vi "initialize.vi"() -> (0 "ErrorOut":errorcluster, 3 "Queues":T1)   [LabVIEW 2019]
uses:
  utilities/Queues.ctl
  GUIVIs/GUIOutput.ctl
  masterVIs/Command.ctl
  MobileAnalyzer/mainVIs/analyzeAccelerationDataVIs/AccelerationDataFrames.ctl
  MobileAnalyzer/mainVIs/analyzeAccelerationDataVIs/AnalyzedVibrationsData.ctl
  MobileAnalyzer/mainVIs/analyzeAccelerationDataVIs/calculateFaultIndicatorsVIs/FaultDetections.ctl
  MobileAnalyzer/mainVIs/analyzeAccelerationDataVIs/calculateFaultIndicatorsVIs/FaultParameter.ctl
  MobileAnalyzer/mainVIs/analyzeAccelerationDataVIs/calculateFaultIndicatorsVIs/AxesValueAndFaultDetection.ctl
  utilities/DesktopAppSettings.ctl
  masterVIs/Thread.ctl
  MobileAnalyzer/mainVIs/analyzeAccelerationDataVIs/calculateFaultIndicatorsVIs/Thresholds.ctl
  MobileAnalyzer/mainVIs/utilities/FGVAction.ctl
  DialogsVIs/FilePathToSaveAction.ctl
  masterVIs/CommandQueuesAction.ctl
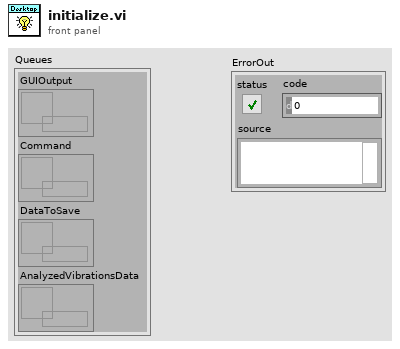
[diagram p1: front panel]
types:
  T1 = typedef "Queues.ctl" = cluster{"GUIOutput":refnum<queue>, "Command":refnum<queue>, "DataToSave":refnum<queue>, "AnalyzedVibrationsData":refnum<queue>}
  T2 = typedef "AnalyzedVibrationsData.ctl" = cluster{"AccelerationDataFrames":T3, "Fault detections":T4}
  T3 = typedef "AccelerationDataFrames.ctl" = cluster{"AccelerationData":waveform(dbl)[], "Amplitudes":cluster{"f0":dbl, "df":dbl, "real part":dbl[]}[], "Phases":cluster{"f0":dbl, "df":dbl, "imaginary part":dbl[]}[]}
  T4 = typedef "FaultDetections.ctl" = cluster{"Parameters labels":T5[], "Parameters fault detection":T6[], "Frequencies fault detection":T6[]}
  T5 = typedef "FaultParameter.ctl" = enum16{"Kurtosis", "RMS"}
  T6 = typedef "AxesValueAndFaultDetection.ctl" = cluster{"Axes Values":dbl[], "Axes Fault Detection":bool[]}
  T7 = typedef "Command.ctl" = enum16{"None", "Connect", "Start", "Stop", "RestartAnalyzer", "Exit", "OpenDataFile", "CanBegin", "FileToSaveSettings", "SetThresholds"}
  T8 = typedef "FilePathToSaveAction.ctl" = enum16{"Build new path", "Update index", "Get file path", "Get current settings"}
  T9 = typedef "FGVAction.ctl" = enum16{"Read", "Write"}
  T10 = typedef "CommandQueuesAction.ctl" = enum16{"Initialize", "Set", "Get", "ReleaseAll"}
  T11 = typedef "GUIOutput.ctl" = cluster{"Aquiring data":bool, "AnalyzerError":errorcluster, "FIFO overflow":bool, "Analyzing data":bool, "Connected":bool}
  T12 = typedef "Thread.ctl" = enum16{"GUI", "communicateWithAnalyzer", "saveDataToTDMS"}
  T13 = typedef "DesktopAppSettings.ctl" = cluster{"MobileAnalyzer IP":string, "Network Stream Timeout Code":i32, "Endpoint Destroyed Code":i32, "Save to file?":bool, "All threads":T12[], "Fault Thresholds":T14}
  T14 = typedef "Thresholds.ctl" = cluster{"Parameters labels":T5[], "Parameters thresholds":dbl[], "Freqs and thresholds":dbl[][]}
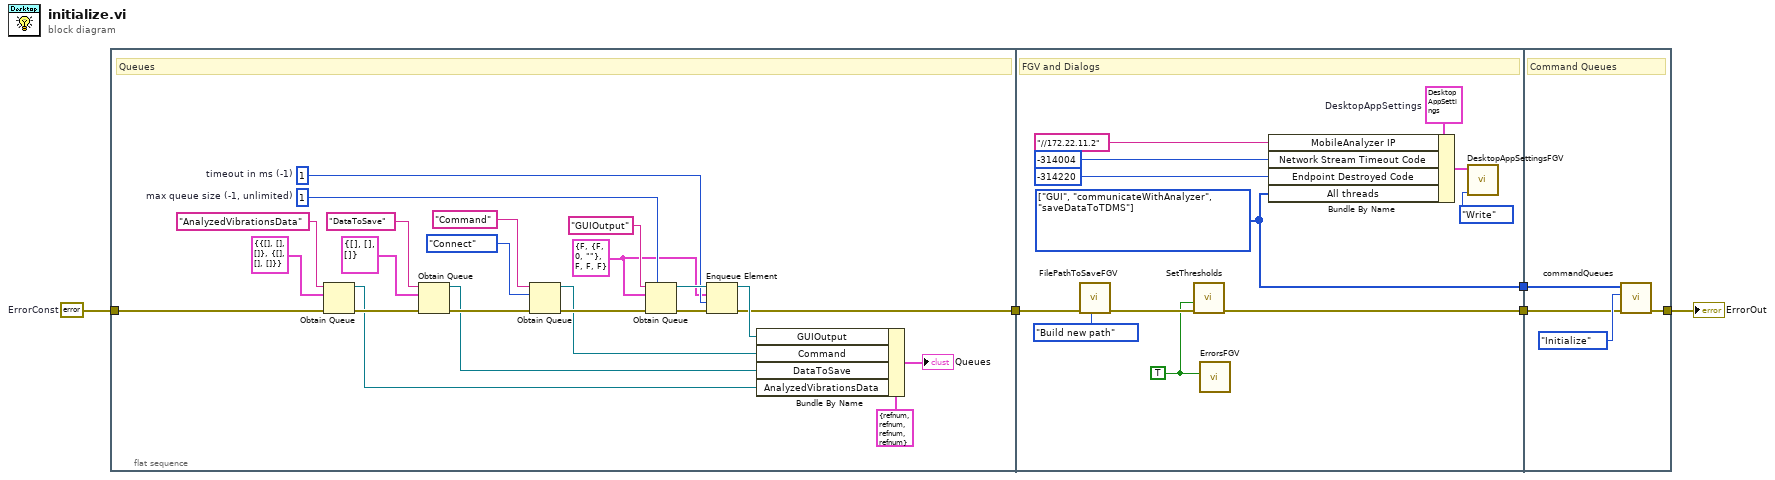
[diagram p0: block diagram]
diagram:
  w5 = errorcluster {"status"=FALSE, "code"=0, "source"=""}  # ErrorConst
  n1 = flat-sequence {
    tunnel: w5 -> [w24]
    tunnel: [w13] -> w3
    tunnel: w3 -> [w33]
    tunnel: [w30] -> w2
    tunnel: [w34] -> w1
    tunnel: [w42] -> w4
    tunnel: w2 -> [w43]
    tunnel: w1 -> [w41]
    frame #0 {
      w18 = T11 {"Aquiring data"=FALSE, "AnalyzerError"={"status"=FALSE, "code"=0, "source"=""}, "FIFO overflow"=FALSE, "Analyzing data"=FALSE, "Connected"=FALSE} ("UIOutput")
      w19 = 1  # timeout in ms (-1)
      w20 = 1  # max queue size (-1, unlimited)
      # "Queues"
      n2 = Obtain Queue(name (unnamed)="AnalyzedVibrationsData", element data type=T2 {"AccelerationDataFrames"={"AccelerationData"=[], "Amplitudes"=[], "Phases"=[]}, "Fault detections"={"Parameters labels"=[], "Parameters fault detection"=[], "Frequencies fault detection"=[]}} ("AnalyzedVibrationsData"), error in (no error)=w24) -> (queue out=w8:refnum<queue>, error out=w12:errorcluster)  [unwired: 2 in, 1 out]
      n3 = Obtain Queue(name (unnamed)="DataToSave", element data type=T3 {"AccelerationData"=[], "Amplitudes"=[], "Phases"=[]} ("AccelerationDataFrames"), error in (no error)=w12) -> (queue out=w7:refnum<queue>, error out=w11:errorcluster)  [unwired: 2 in, 1 out]
      n4 = Obtain Queue(name (unnamed)="Command", element data type=Command."Connect" ("Command"), error in (no error)=w11) -> (queue out=w14:refnum<queue>, error out=w27:errorcluster)  [unwired: 2 in, 1 out]
      n5 = Obtain Queue(max queue size (-1, unlimited)=w20, name (unnamed)="GUIOutput" ("writer name"), element data type=w18, error in (no error)=w27) -> (queue out=w22:refnum<queue>, error out=w23:errorcluster)  [unwired: 1 in, 1 out]
      n6 = Enqueue Element(queue=w22, element=w18, timeout in ms (-1)=w19, error in (no error)=w23) -> (queue out=w17:refnum<queue>, error out=w13:errorcluster)  [unwired: 1 out]
      n7 = Bundle By Name(cluster=T1 {"GUIOutput"=refnum, "Command"=refnum, "DataToSave"=refnum, "AnalyzedVibrationsData"=refnum} ("Queues"), "GUIOutput"=w17, "Command"=w14, "DataToSave"=w7, "AnalyzedVibrationsData"=w8) -> (→"Queues":T1)
    }
    frame #1 {
      w34 = T12[] [enum."GUI", enum."communicateWithAnalyzer", enum."saveDataToTDMS"] items=["GUI", "communicateWithAnalyzer", "saveDataToTDMS"] ("Threads")
      w29 = TRUE ("Reset?")
      w40 = T13 {"MobileAnalyzer IP"="//172.22.11.2", "Network Stream Timeout Code"=-314004, "Endpoint Destroyed Code"=0, "Save to file?"=FALSE, "All threads"=[], "Fault Thresholds"={"Parameters labels"=[], "Parameters thresholds"=[], "Freqs and thresholds"=[]}}  # DesktopAppSettings
      # "FGV and Dialogs"
      n8 = call "FilePathToSaveFGV.vi"("FilePathToSaveAction"=FilePathToSaveAction."Build new path", "ErrorIn"=w33) -> ("ErrorOut"=w31:errorcluster)  [unwired: 6 in, 3 out]
      n9 = call "SetThresholds.vi"("ErrorIn"=w31, "Set default thresholds? [F]"=w29) -> ("ErrorOut"=w30:errorcluster)  [unwired: 9 in]
      n10 = call "ErrorsFGV.vi"("Reset?"=w29) -> ()  [unwired: 7 in, 4 out]
      n11 = Bundle By Name(cluster=w40, "MobileAnalyzer IP"="//172.22.11.2", "Network Stream Timeout Code"=-314004, "Endpoint Destroyed Code"=-314220, "All threads"=w34) -> (w39:T13)
      n12 = call "DesktopAppSettingsFGV.vi"("FGVAction (Read)"=FGVAction."Write", "DesktopAppSettingsIn"=w39) -> ()  [unwired: 9 in, 1 out]
    }
    frame #2 {
      # "Command Queues"
      n13 = call "commandQueues.vi"("ErrorIn"=w43, "CommandQueuesAction"=CommandQueuesAction."Initialize", "Threads"=w41) -> ("ErrorOut"=w42:errorcluster)  [unwired: 7 in, 1 out]
    }
  }
  "ErrorOut" <- w4
